vi "GetParam.vi"(8 "error in (no error)":errorcluster caption="entrée d'erreur (pas d'erreur)", 11 "Mean_Gamma_Deviance.lvclass":refnum<class "Mean_Gamma_Deviance.lvclass">) -> (0 "error out":errorcluster caption="sortie d'erreur", 2 "mean_gamma_deviance":cluster{"sample_weight":dbl[]}, 3 "Mean_Gamma_Deviance.lvclass":refnum<class "Mean_Gamma_Deviance.lvclass">)   [LabVIEW 2020, in "Mean_Gamma_Deviance.lvclass"]
doc: "Get Parameters"
uses:
  Mean_Gamma_Deviance.lvclass
  Mean_Gamma_Deviance.lvclass/Mean_Gamma_Deviance.ctl
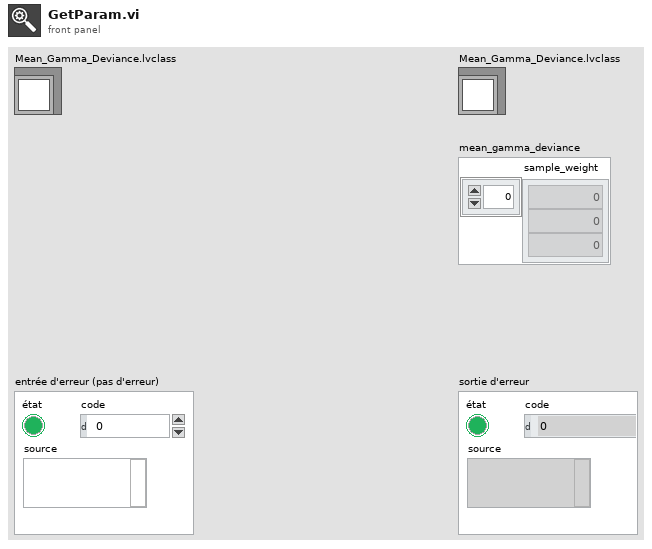
[diagram p1: front panel]
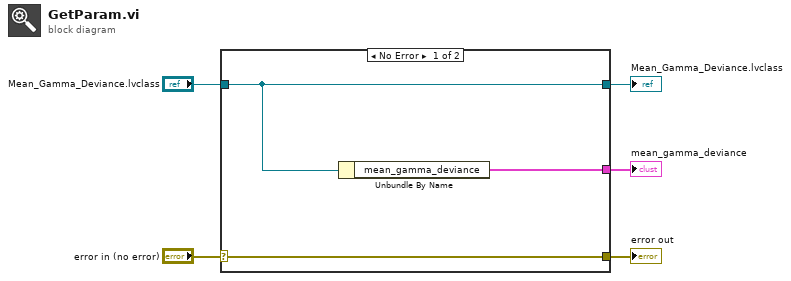
[diagram p0: block diagram]
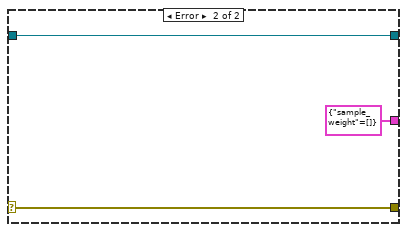
[diagram p2: hidden frame]
diagram:
  n1 = case shown="No Error" "error in (no error)" {
    selector: "error in (no error)" -> [w8 w10]
    tunnel: [w8 w10] -> w4
    tunnel: [w7 w11] -> w2
    tunnel: "Mean_Gamma_Deviance.lvclass" -> [w7 w11]
    tunnel: [w6 cluster{"sample_weight":dbl[]} {"sample_weight"=[]} ("mean_gamma_deviance")] -> w1
    frame No Error {
      n2 = Unbundle By Name(w7) -> ("mean_gamma_deviance"=w6:cluster{"sample_weight":dbl[]})
    }
    frame Error {
    }
  }
  "error out" <- w4
  "Mean_Gamma_Deviance.lvclass" <- w2
  "mean_gamma_deviance" <- w1
